vi "CheckWin.vi"(1 "place":i32, 2 "player":i32, 3 "Board":i32[][](array[numeric])) -> (0 "win":bool)   [LabVIEW 2025]
panel:
  out "row":i32
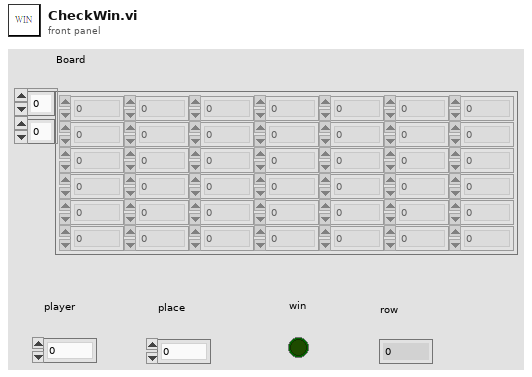
[diagram p1: front panel]
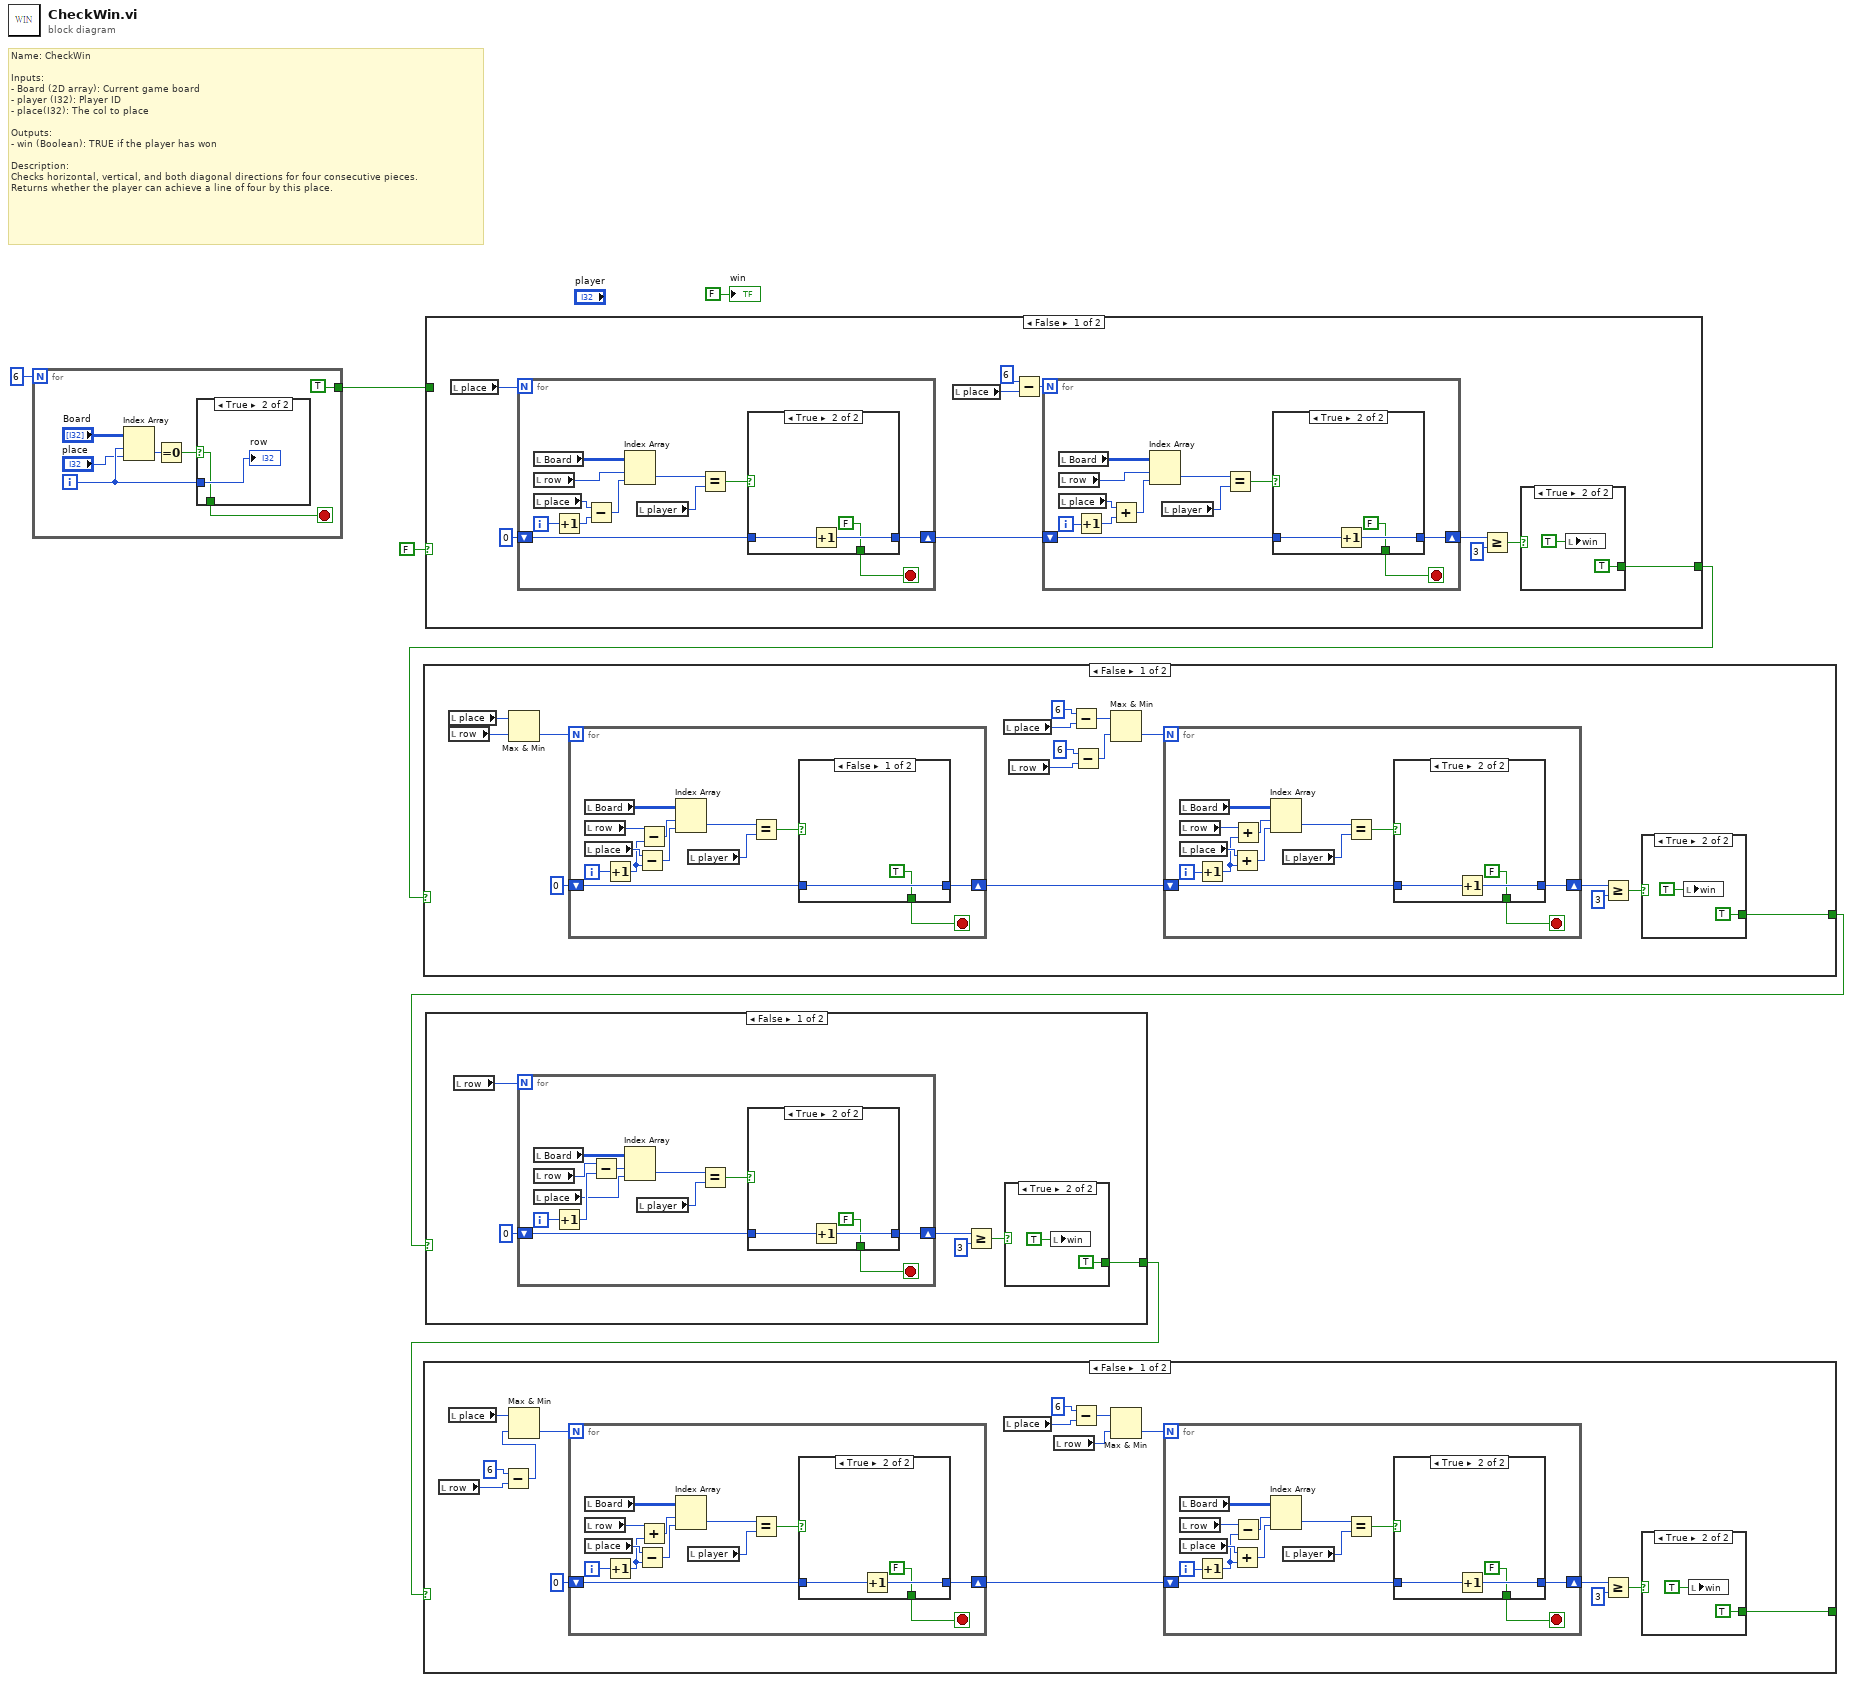
[diagram p0: block diagram]
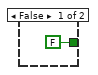
[diagram p2: hidden frame]
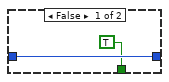
[diagram p3: hidden frame]
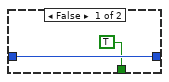
[diagram p4: hidden frame]
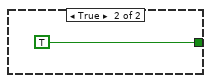
[diagram p5: hidden frame]
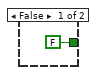
[diagram p6: hidden frame]
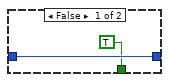
[diagram p7: hidden frame]
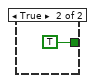
[diagram p8: hidden frame]
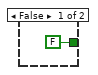
[diagram p9: hidden frame]
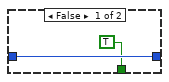
[diagram p10: hidden frame]
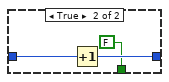
[diagram p11: hidden frame]
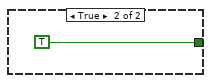
[diagram p12: hidden frame]
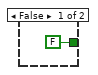
[diagram p14: hidden frame]
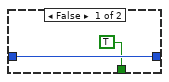
[diagram p15: hidden frame]
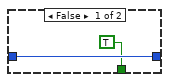
[diagram p16: hidden frame]
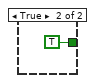
[diagram p17: hidden frame]
diagram:
  # "Name: CheckWin\n\nInputs:\n- Board (2D array): Current game board\n- player (I32): Player ID\n- place(I32): The col to place\n\nOutputs:\n- win (Boolean): TRUE if the player has won\n\nDescription:\nChecks horizontal, vertical, and both diagonal directions for four consecutive pieces.\nReturns whether the player can achieve a line of four by this place."
  n1 = for {
    N: 6 -> [_]
    tunnel: [TRUE] -> w5
    i -> [w9]
    stop <- w11 stop-if-true
    n2 = Index Array(array="Board", index (row)=w9, index (col)="place") -> (element=w12:i32)
    n3 = Equal To 0?(x=w12) -> (x = 0?=w14:bool)
    n4 = case shown="True" w14 {
      selector: w14 -> [w15 w16]
      tunnel: w9 -> [_ w17]
      tunnel: [w15 w16] -> w11
      frame False {
      }
      frame True {
        "row" <- w17
      }
    }
  }
  n5 = case shown="False" FALSE {
    tunnel: w5 -> [_ _]
    tunnel: [w18 TRUE] -> w3
    frame False {
      n6 = local read "place"() -> (w26:i32)
      n7 = for {
        N: w26 -> [_]
        shift-right: [w52] -> w25
        shift-left: 0 -> [w51]
        i -> [w49]
        stop <- w50 stop-if-true
        n8 = local read "Board"() -> (w59:i32[][])
        n9 = local read "row"() -> (w56:i32)
        n10 = local read "place"() -> (w58:i32)
        n11 = Increment(x=w49) -> (x+1=w48:i32)
        n12 = Subtract(x=w58, y=w48) -> (x-y=w57:i32)
        n13 = Index Array(array=w59, index (row)=w56, index (col)=w57) -> (element=w55:i32)
        n14 = local read "player"() -> (w54:i32)
        n15 = Equal?(x=w55, y=w54) -> (x = y?=w53:bool)
        n16 = case shown="True" w53 {
          tunnel: [w61 w64] -> w52
          tunnel: w51 -> [w61 w63]
          tunnel: [TRUE FALSE] -> w50
          frame False {
          }
          frame True {
            n17 = Increment(x=w63) -> (x+1=w64:i32)
          }
        }
      }
      n18 = local read "place"() -> (w23:i32)
      n19 = Subtract(x=6, y=w23) -> (x-y=w24:i32)
      n20 = for {
        N: w24 -> [_]
        shift-right: [w35] -> w21
        shift-left: w25 -> [w34]
        i -> [w32]
        stop <- w33 stop-if-true
        n21 = local read "Board"() -> (w42:i32[][])
        n22 = local read "row"() -> (w39:i32)
        n23 = local read "place"() -> (w41:i32)
        n24 = Increment(x=w32) -> (x+1=w31:i32)
        n25 = Add(x=w41, y=w31) -> (x+y=w40:i32)
        n26 = Index Array(array=w42, index (row)=w39, index (col)=w40) -> (element=w38:i32)
        n27 = local read "player"() -> (w37:i32)
        n28 = Equal?(x=w38, y=w37) -> (x = y?=w36:bool)
        n29 = case shown="True" w36 {
          tunnel: [w44 w47] -> w35
          tunnel: w34 -> [w44 w46]
          tunnel: [TRUE FALSE] -> w33
          frame False {
          }
          frame True {
            n30 = Increment(x=w46) -> (x+1=w47:i32)
          }
        }
      }
      n31 = Greater Or Equal?(x=w21, y=3) -> (x >= y?=w19:bool)
      n32 = case shown="True" w19 {
        tunnel: [FALSE TRUE] -> w18
        frame False {
        }
        frame True {
          n33 = local write "win"(TRUE ("win")) -> ()
        }
      }
    }
    frame True {
    }
  }
  n34 = case shown="False" w3 {
    tunnel: [w66 TRUE] -> w1
    frame False {
      n35 = local read "place"() -> (w75:i32)
      n36 = local read "row"() -> (w74:i32)
      n37 = Max & Min(x=w75, y=w74) -> (min(x,y)=w76:i32)  [unwired: 1 out]
      n38 = for {
        N: w76 -> [_]
        shift-right: [w109] -> w80
        shift-left: 0 -> [w108]
        i -> [w106]
        stop <- w107 stop-if-true
        n39 = local read "Board"() -> (w115:i32[][])
        n40 = local read "row"() -> (w105:i32)
        n41 = local read "place"() -> (w114:i32)
        n42 = Increment(x=w106) -> (x+1=w103:i32)
        n43 = Subtract(x=w114, y=w103) -> (x-y=w113:i32)
        n44 = Subtract(x=w105, y=w103) -> (x-y=w104:i32)
        n45 = Index Array(array=w115, index (row)=w104, index (col)=w113) -> (element=w112:i32)
        n46 = local read "player"() -> (w111:i32)
        n47 = Equal?(x=w112, y=w111) -> (x = y?=w110:bool)
        n48 = case shown="False" w110 {
          tunnel: [w117 w120] -> w109
          tunnel: w108 -> [w117 w119]
          tunnel: [TRUE FALSE] -> w107
          frame False {
          }
          frame True {
            n49 = Increment(x=w119) -> (x+1=w120:i32)
          }
        }
      }
      n50 = local read "place"() -> (w72:i32)
      n51 = local read "row"() -> (w71:i32)
      n52 = Subtract(x=6, y=w72) -> (x-y=w68:i32)
      n53 = Subtract(x=6, y=w71) -> (x-y=w67:i32)
      n54 = Max & Min(x=w68, y=w67) -> (min(x,y)=w69:i32)  [unwired: 1 out]
      n55 = for {
        N: w69 -> [_]
        shift-right: [w92] -> w79
        shift-left: w80 -> [w85]
        i -> [w90]
        stop <- w91 stop-if-true
        n56 = local read "Board"() -> (w97:i32[][])
        n57 = local read "row"() -> (w86:i32)
        n58 = local read "place"() -> (w96:i32)
        n59 = Increment(x=w90) -> (x+1=w87:i32)
        n60 = Add(x=w96, y=w87) -> (x+y=w89:i32)
        n61 = Add(x=w86, y=w87) -> (x+y=w88:i32)
        n62 = Index Array(array=w97, index (row)=w88, index (col)=w89) -> (element=w95:i32)
        n63 = local read "player"() -> (w94:i32)
        n64 = Equal?(x=w95, y=w94) -> (x = y?=w93:bool)
        n65 = case shown="True" w93 {
          tunnel: [w99 w102] -> w92
          tunnel: w85 -> [w99 w101]
          tunnel: [TRUE FALSE] -> w91
          frame False {
          }
          frame True {
            n66 = Increment(x=w101) -> (x+1=w102:i32)
          }
        }
      }
      n67 = Greater Or Equal?(x=w79, y=3) -> (x >= y?=w77:bool)
      n68 = case shown="True" w77 {
        tunnel: [FALSE TRUE] -> w66
        frame False {
        }
        frame True {
          n69 = local write "win"(TRUE ("win")) -> ()
        }
      }
    }
    frame True {
    }
  }
  n70 = case shown="False" w1 {
    tunnel: [w123 TRUE] -> w2
    frame False {
      n71 = local read "row"() -> (w126:i32)
      n72 = for {
        N: w126 -> [_]
        shift-right: [w138] -> w122
        shift-left: 0 -> [w137]
        i -> [w135]
        stop <- w136 stop-if-true
        n73 = local read "Board"() -> (w142:i32[][])
        n74 = local read "row"() -> (w133:i32)
        n75 = local read "place"() -> (w131:i32)
        n76 = Increment(x=w135) -> (x+1=w134:i32)
        n77 = Subtract(x=w133, y=w134) -> (x-y=w132:i32)
        n78 = Index Array(array=w142, index (row)=w132, index (col)=w131) -> (element=w141:i32)
        n79 = local read "player"() -> (w140:i32)
        n80 = Equal?(x=w141, y=w140) -> (x = y?=w139:bool)
        n81 = case shown="True" w139 {
          tunnel: [w144 w147] -> w138
          tunnel: w137 -> [w144 w146]
          tunnel: [TRUE FALSE] -> w136
          frame False {
          }
          frame True {
            n82 = Increment(x=w146) -> (x+1=w147:i32)
          }
        }
      }
      n83 = Greater Or Equal?(x=w122, y=3) -> (x >= y?=w124:bool)
      n84 = case shown="True" w124 {
        tunnel: [FALSE TRUE] -> w123
        frame False {
        }
        frame True {
          n85 = local write "win"(TRUE ("win")) -> ()
        }
      }
    }
    frame True {
    }
  }
  n86 = case shown="False" w2 {
    tunnel: [w153 TRUE] -> _
    frame False {
      n87 = local read "row"() -> (w151:i32)
      n88 = local read "place"() -> (w158:i32)
      n89 = Subtract(x=6, y=w151) -> (x-y=w150:i32)
      n90 = Max & Min(x=w158, y=w150) -> (min(x,y)=w159:i32)  [unwired: 1 out]
      n91 = for {
        N: w159 -> [_]
        shift-right: [w192] -> w163
        shift-left: 0 -> [w191]
        i -> [w189]
        stop <- w190 stop-if-true
        n92 = local read "Board"() -> (w198:i32[][])
        n93 = local read "row"() -> (w188:i32)
        n94 = local read "place"() -> (w197:i32)
        n95 = Increment(x=w189) -> (x+1=w186:i32)
        n96 = Subtract(x=w197, y=w186) -> (x-y=w196:i32)
        n97 = Add(x=w188, y=w186) -> (x+y=w187:i32)
        n98 = Index Array(array=w198, index (row)=w187, index (col)=w196) -> (element=w195:i32)
        n99 = local read "player"() -> (w194:i32)
        n100 = Equal?(x=w195, y=w194) -> (x = y?=w193:bool)
        n101 = case shown="True" w193 {
          tunnel: [w200 w203] -> w192
          tunnel: w191 -> [w200 w202]
          tunnel: [TRUE FALSE] -> w190
          frame False {
          }
          frame True {
            n102 = Increment(x=w202) -> (x+1=w203:i32)
          }
        }
      }
      n103 = local read "place"() -> (w156:i32)
      n104 = local read "row"() -> (w149:i32)
      n105 = Subtract(x=6, y=w156) -> (x-y=w154:i32)
      n106 = Max & Min(x=w154, y=w149) -> (min(x,y)=w155:i32)  [unwired: 1 out]
      n107 = for {
        N: w155 -> [_]
        shift-right: [w175] -> w162
        shift-left: w163 -> [w168]
        i -> [w173]
        stop <- w174 stop-if-true
        n108 = local read "Board"() -> (w180:i32[][])
        n109 = local read "row"() -> (w169:i32)
        n110 = local read "place"() -> (w179:i32)
        n111 = Increment(x=w173) -> (x+1=w170:i32)
        n112 = Add(x=w179, y=w170) -> (x+y=w172:i32)
        n113 = Subtract(x=w169, y=w170) -> (x-y=w171:i32)
        n114 = Index Array(array=w180, index (row)=w171, index (col)=w172) -> (element=w178:i32)
        n115 = local read "player"() -> (w177:i32)
        n116 = Equal?(x=w178, y=w177) -> (x = y?=w176:bool)
        n117 = case shown="True" w176 {
          tunnel: [w182 w185] -> w175
          tunnel: w168 -> [w182 w184]
          tunnel: [TRUE FALSE] -> w174
          frame False {
          }
          frame True {
            n118 = Increment(x=w184) -> (x+1=w185:i32)
          }
        }
      }
      n119 = Greater Or Equal?(x=w162, y=3) -> (x >= y?=w160:bool)
      n120 = case shown="True" w160 {
        tunnel: [FALSE TRUE] -> w153
        frame False {
        }
        frame True {
          n121 = local write "win"(TRUE ("win")) -> ()
        }
      }
    }
    frame True {
    }
  }
  "win" <- FALSE ("win")
